vi "ShowErrorDLVI.vi"(8 "error in (no error)":errorcluster, 11 "DelayLine in":refnum<class "DelayLine.lvclass">) -> (0 "error out":errorcluster, 3 "DelayLine out":refnum<class "DelayLine.lvclass">)   [LabVIEW 2015, in "DelayLine.lvclass"]
uses:
  DelayLine.lvclass
  GeneralFunctionality/GeneralFunctionality.lvclass/GeneralFunctionality.ctl
  GeneralFunctionality/GeneralFunctionality.lvclass
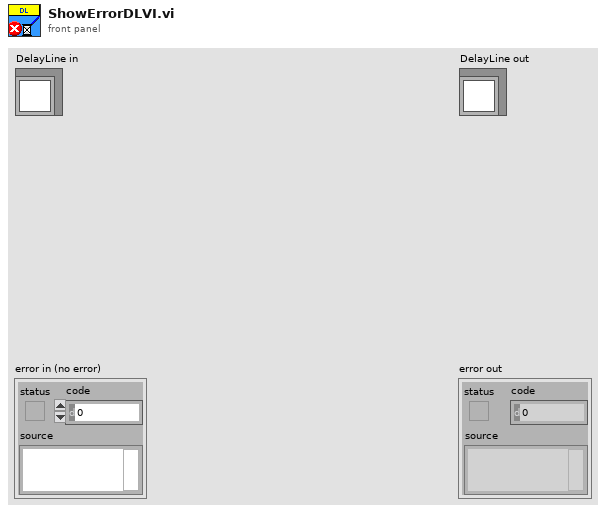
[diagram p1: front panel]
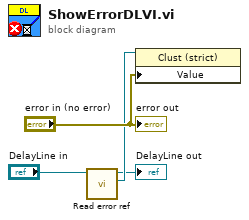
[diagram p0: block diagram]
diagram:
  n1 = call "Read error ref.vi"("GeneralFunctionality in"="DelayLine in") -> ("error"=w2:refnum<vi>, "GeneralFunctionality out"=→"DelayLine out":refnum<class "DelayLine.lvclass">)  [unwired: 8 in, 1 out]
  n2 = property class="Clust (strict)"(reference=w2, "Value"="error in (no error)") -> ()  [unwired: 1 in, 2 out]
  "error out" <- "error in (no error)"
